vi "Get Enumerator.vi"(8 "error in (no error)":errorcluster caption="错误输入（无错误）", 11 "Stack 输入":refnum<class "Stack.lvclass"> caption="DNL_LabVIEW Object in") -> (0 "error out":errorcluster caption="错误输出", 2 "Enumerator 输出":refnum<class "Enumerator.lvclass">, 3 "Stack 输出":refnum<class "Stack.lvclass"> caption="DNL_LabVIEW Object out")   [LabVIEW 2011, in "Stack.lvclass"]
uses:
  Stack.lvclass
  Enumerator/Enumerator.lvclass
  Stack.lvclass/Stack.ctl
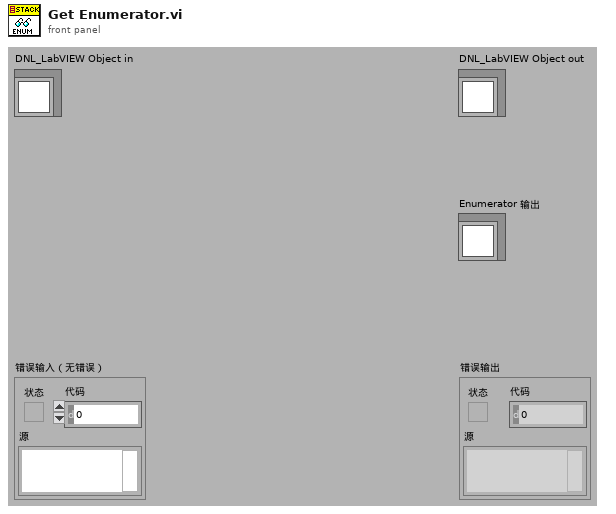
[diagram p1: front panel]
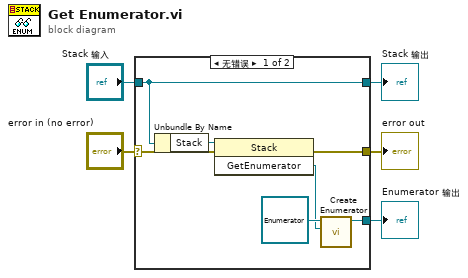
[diagram p0: block diagram]
diagram:
  n1 = case shown="无错误" "error in (no error)" {
    selector: "error in (no error)" -> [w7 w14]
    tunnel: [w6 w14] -> w4
    tunnel: [w12 w13] -> w2
    tunnel: "Stack 输入" -> [w12 w13]
    tunnel: [w8 _] -> w1
    frame No Error {
      n2 = Unbundle By Name(w12) -> ("Stack"=w11:refnum<k24>)
      n3 = invoke class="Stack" method="GetEnumerator"(reference=w11, error in=w7) -> (error out=w6:errorcluster, "GetEnumerator"=w9:refnum<k24>)  [unwired: 1 in, 1 out]
      n4 = call "Create Enumerator.vi"("Enumerator"=w9, "Enumerator 输入"=refnum<class "Enumerator.lvclass"> refnum ("Enumerator.lvclass")) -> ("Enumerator 输出"=w8:refnum<class "Enumerator.lvclass">)  [unwired: 8 in, 1 out]
    }
    frame Error {
    }
  }
  "error out" <- w4
  "Stack 输出" <- w2
  "Enumerator 输出" <- w1
